vi "BuildRX.vi"() -> (0 "RX":bool[][](array[boolean]))   [LabVIEW 2018]
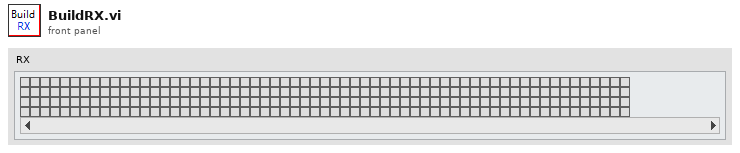
[diagram p1: front panel]
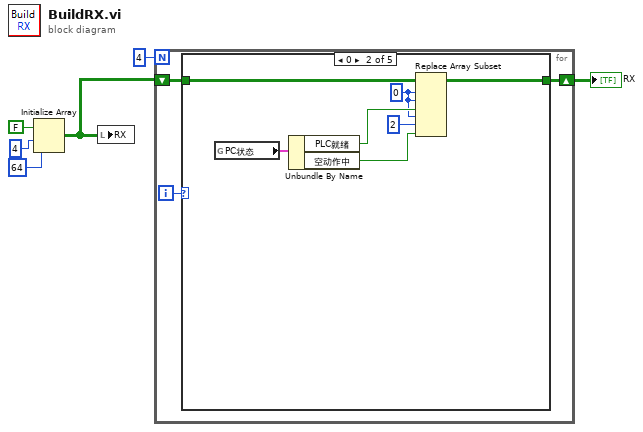
[diagram p0: block diagram]
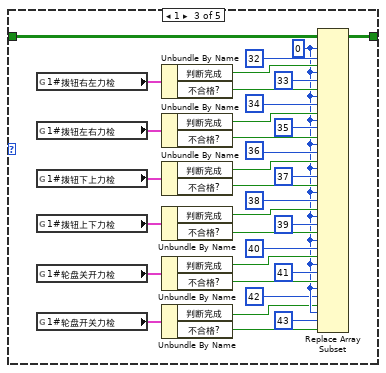
[diagram p3: hidden frame]
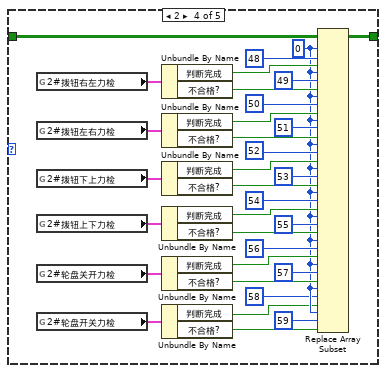
[diagram p4: hidden frame]
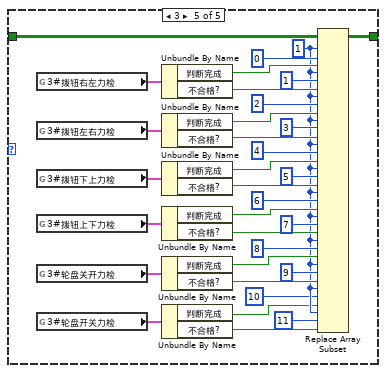
[diagram p5: hidden frame]
diagram:
  n1 = Initialize Array(FALSE, 4 ("维数大小"), 64 ("维数大小")) -> (w6:bool[][])
  n2 = local write "RX"(w6) -> ()
  n3 = for {
    N: 4 -> [_]
    shift-right: [w7] -> w1
    shift-left: w6 -> [w8]
    i -> [w9]
    n4 = case shown="0" w9 {
      tunnel: w8 -> [w10 w16 w49 w82 w115]
      tunnel: [w10 w11 w45 w78 w111] -> w7
      frame -1, Default {
      }
      frame 0 {
        w14 = 0 ("索引 (行)")
        n5 = global read "全局 1.vi" "PC状态"() -> (w17:cluster{"PLC就绪":bool, "空动作中":bool})
        n6 = Unbundle By Name(w17) -> ("PLC就绪"=w15:bool, "空动作中"=w12:bool)
        n7 = Replace Array Subset(array=w16, new element #1=w15, index (row) #1=w14, index (col) #1=w14, new element #2=w12, index (row) #2=w14, index (col) #2=2 ("禁用的索引 (列)")) -> (w11:bool[][])
      }
      frame 1 {
        w23 = 0 ("索引 (行)")
        n8 = global read "全局F结果.vi" "1#拨钮右左力检"() -> (w50:cluster{"判断完成":bool, "不合格?":bool})
        n9 = global read "全局F结果.vi" "1#拨钮左右力检"() -> (w43:cluster{"判断完成":bool, "不合格?":bool})
        n10 = global read "全局F结果.vi" "1#拨钮下上力检"() -> (w38:cluster{"判断完成":bool, "不合格?":bool})
        n11 = global read "全局F结果.vi" "1#拨钮上下力检"() -> (w33:cluster{"判断完成":bool, "不合格?":bool})
        n12 = global read "全局F结果.vi" "1#轮盘关开力检"() -> (w28:cluster{"判断完成":bool, "不合格?":bool})
        n13 = global read "全局F结果.vi" "1#轮盘开关力检"() -> (w20:cluster{"判断完成":bool, "不合格?":bool})
        n14 = Unbundle By Name(w50) -> ("判断完成"=w48:bool, "不合格?"=w46:bool)
        n15 = Unbundle By Name(w43) -> ("判断完成"=w40:bool, "不合格?"=w39:bool)
        n16 = Unbundle By Name(w38) -> ("判断完成"=w35:bool, "不合格?"=w34:bool)
        n17 = Unbundle By Name(w33) -> ("判断完成"=w29:bool, "不合格?"=w30:bool)
        n18 = Unbundle By Name(w28) -> ("判断完成"=w25:bool, "不合格?"=w24:bool)
        n19 = Unbundle By Name(w20) -> ("判断完成"=w18:bool, "不合格?"=w19:bool)
        n20 = Replace Array Subset(array=w49, new element #1=w48, index (row) #1=w23, index (col) #1=32 ("索引 (行)"), new element #2=w46, index (row) #2=w23, index (col) #2=33 ("禁用的索引 (列)"), new element #3=w40, index (row) #3=w23, index (col) #3=34 ("索引 (行)"), new element #4=w39, index (row) #4=w23, index (col) #4=35 ("禁用的索引 (列)"), new element #5=w35, index (row) #5=w23, index (col) #5=36 ("索引 (行)"), new element #6=w34, index (row) #6=w23, index (col) #6=37 ("禁用的索引 (列)"), new element #7=w29, index (row) #7=w23, index (col) #7=38 ("索引 (行)"), new element #8=w30, index (row) #8=w23, index (col) #8=39 ("禁用的索引 (列)"), new element #9=w25, index (row) #9=w23, index (col) #9=40 ("索引 (行)"), new element #10=w24, index (row) #10=w23, index (col) #10=41 ("禁用的索引 (列)"), new element #11=w18, index (row) #11=w23, index (col) #11=42 ("索引 (行)"), new element #12=w19, index (row) #12=w23, index (col) #12=43 ("禁用的索引 (列)")) -> (w45:bool[][])
      }
      frame 2 {
        w56 = 0 ("索引 (行)")
        n21 = global read "全局F结果.vi" "2#拨钮右左力检"() -> (w83:cluster{"判断完成":bool, "不合格?":bool})
        n22 = global read "全局F结果.vi" "2#拨钮左右力检"() -> (w76:cluster{"判断完成":bool, "不合格?":bool})
        n23 = global read "全局F结果.vi" "2#拨钮下上力检"() -> (w71:cluster{"判断完成":bool, "不合格?":bool})
        n24 = global read "全局F结果.vi" "2#拨钮上下力检"() -> (w66:cluster{"判断完成":bool, "不合格?":bool})
        n25 = global read "全局F结果.vi" "2#轮盘关开力检"() -> (w61:cluster{"判断完成":bool, "不合格?":bool})
        n26 = global read "全局F结果.vi" "2#轮盘开关力检"() -> (w53:cluster{"判断完成":bool, "不合格?":bool})
        n27 = Unbundle By Name(w83) -> ("判断完成"=w81:bool, "不合格?"=w79:bool)
        n28 = Unbundle By Name(w76) -> ("判断完成"=w73:bool, "不合格?"=w72:bool)
        n29 = Unbundle By Name(w71) -> ("判断完成"=w68:bool, "不合格?"=w67:bool)
        n30 = Unbundle By Name(w66) -> ("判断完成"=w62:bool, "不合格?"=w63:bool)
        n31 = Unbundle By Name(w61) -> ("判断完成"=w58:bool, "不合格?"=w57:bool)
        n32 = Unbundle By Name(w53) -> ("判断完成"=w51:bool, "不合格?"=w52:bool)
        n33 = Replace Array Subset(array=w82, new element #1=w81, index (row) #1=w56, index (col) #1=48 ("索引 (行)"), new element #2=w79, index (row) #2=w56, index (col) #2=49 ("禁用的索引 (列)"), new element #3=w73, index (row) #3=w56, index (col) #3=50 ("索引 (行)"), new element #4=w72, index (row) #4=w56, index (col) #4=51 ("禁用的索引 (列)"), new element #5=w68, index (row) #5=w56, index (col) #5=52 ("索引 (行)"), new element #6=w67, index (row) #6=w56, index (col) #6=53 ("禁用的索引 (列)"), new element #7=w62, index (row) #7=w56, index (col) #7=54 ("索引 (行)"), new element #8=w63, index (row) #8=w56, index (col) #8=55 ("禁用的索引 (列)"), new element #9=w58, index (row) #9=w56, index (col) #9=56 ("索引 (行)"), new element #10=w57, index (row) #10=w56, index (col) #10=57 ("禁用的索引 (列)"), new element #11=w51, index (row) #11=w56, index (col) #11=58 ("索引 (行)"), new element #12=w52, index (row) #12=w56, index (col) #12=59 ("禁用的索引 (列)")) -> (w78:bool[][])
      }
      frame 3 {
        w89 = 1 ("索引 (行)")
        n34 = global read "全局F结果.vi" "3#拨钮右左力检"() -> (w116:cluster{"判断完成":bool, "不合格?":bool})
        n35 = global read "全局F结果.vi" "3#拨钮左右力检"() -> (w109:cluster{"判断完成":bool, "不合格?":bool})
        n36 = global read "全局F结果.vi" "3#拨钮下上力检"() -> (w104:cluster{"判断完成":bool, "不合格?":bool})
        n37 = global read "全局F结果.vi" "3#拨钮上下力检"() -> (w99:cluster{"判断完成":bool, "不合格?":bool})
        n38 = global read "全局F结果.vi" "3#轮盘关开力检"() -> (w94:cluster{"判断完成":bool, "不合格?":bool})
        n39 = global read "全局F结果.vi" "3#轮盘开关力检"() -> (w86:cluster{"判断完成":bool, "不合格?":bool})
        n40 = Unbundle By Name(w116) -> ("判断完成"=w114:bool, "不合格?"=w112:bool)
        n41 = Unbundle By Name(w109) -> ("判断完成"=w106:bool, "不合格?"=w105:bool)
        n42 = Unbundle By Name(w104) -> ("判断完成"=w101:bool, "不合格?"=w100:bool)
        n43 = Unbundle By Name(w99) -> ("判断完成"=w95:bool, "不合格?"=w96:bool)
        n44 = Unbundle By Name(w94) -> ("判断完成"=w91:bool, "不合格?"=w90:bool)
        n45 = Unbundle By Name(w86) -> ("判断完成"=w84:bool, "不合格?"=w85:bool)
        n46 = Replace Array Subset(array=w115, new element #1=w114, index (row) #1=w89, index (col) #1=0 ("索引 (行)"), new element #2=w112, index (row) #2=w89, index (col) #2=1 ("禁用的索引 (列)"), new element #3=w106, index (row) #3=w89, index (col) #3=2 ("索引 (行)"), new element #4=w105, index (row) #4=w89, index (col) #4=3 ("禁用的索引 (列)"), new element #5=w101, index (row) #5=w89, index (col) #5=4 ("索引 (行)"), new element #6=w100, index (row) #6=w89, index (col) #6=5 ("禁用的索引 (列)"), new element #7=w95, index (row) #7=w89, index (col) #7=6 ("索引 (行)"), new element #8=w96, index (row) #8=w89, index (col) #8=7 ("禁用的索引 (列)"), new element #9=w91, index (row) #9=w89, index (col) #9=8 ("索引 (行)"), new element #10=w90, index (row) #10=w89, index (col) #10=9 ("禁用的索引 (列)"), new element #11=w84, index (row) #11=w89, index (col) #11=10 ("索引 (行)"), new element #12=w85, index (row) #12=w89, index (col) #12=11 ("禁用的索引 (列)")) -> (w111:bool[][])
      }
    }
  }
  "RX" <- w1
